vi "PositionToCVT.vi"(8 "error in (no error)":errorcluster, 9 "Position Array":dbl[](array[numeric]), 11 "Connected Axes":string[](array[string])) -> (0 "error out":errorcluster)   [LabVIEW 2020]
uses:
  shared/CompressAndUpdate(Poly)/CompressAndUpdate(Numeric).vi
panel:
  out "Variable to update":string
  out "Value":dbl
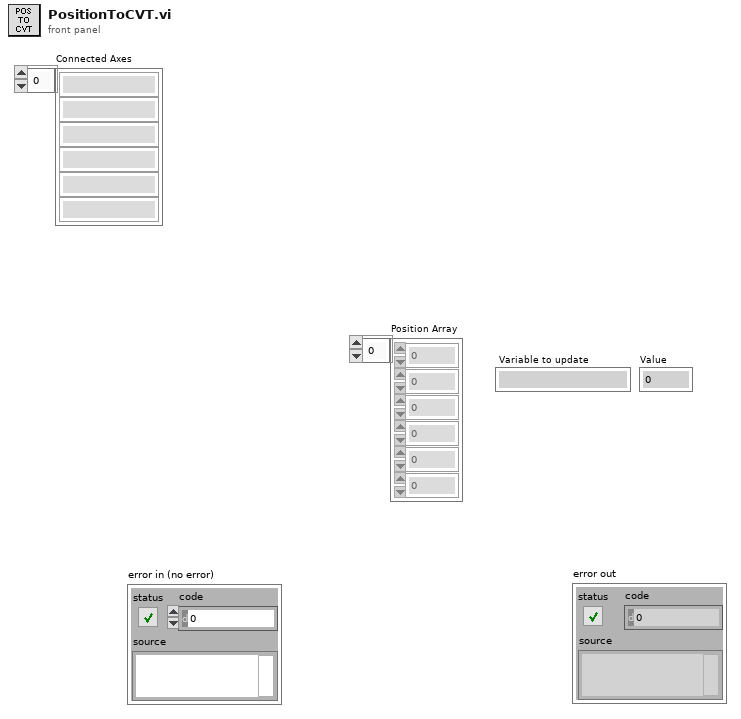
[diagram p1: front panel]
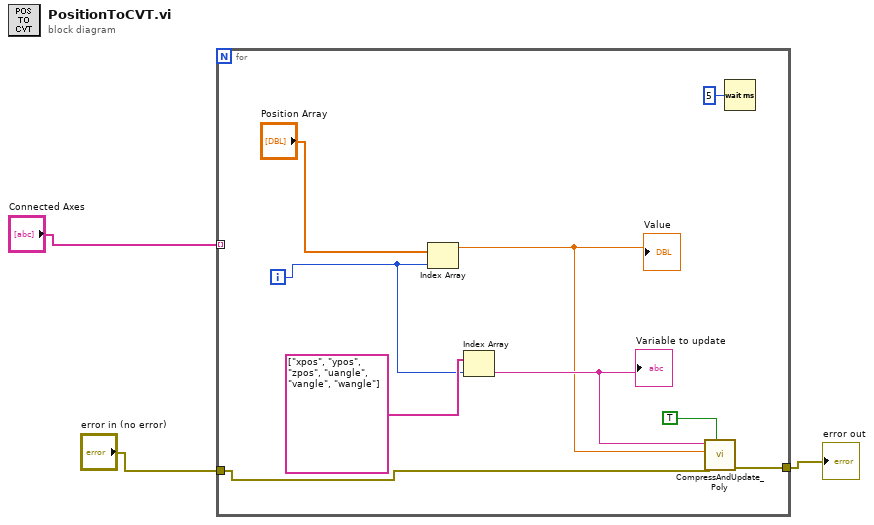
[diagram p0: block diagram]
diagram:
  n1 = for {
    tunnel: "Connected Axes" -> [_] mode=indexing
    tunnel: [w5] -> w1
    tunnel: "error in (no error)" -> [w4]
    i -> [w10]
    n2 = Index Array(array="Position Array", index=w10) -> (element=w7:dbl)
    "Value" <- w7
    n3 = Index Array(array=string[] ["xpos", "ypos", "zpos", "uangle", "vangle", "wangle"], index=w10) -> (element=w8:string)
    "Variable to update" <- w8
    n4 = call-poly "CompressAndUpdate_Poly.vi"("force CVT update (false)"=TRUE, "error in"=w4, "Numeric"=w7, "command or variable name"=w8) -> ("error out"=w5:errorcluster)  [unwired: 7 in]
    n5 = Wait (ms)(milliseconds to wait=u32 5) -> ()  [unwired: 1 out]
  }
  "error out" <- w1
